vi "util_SwitchableDevice_cls_Turn On.vi"(0 "Interface_object in":refnum<class>, 5 "error in (no error)":errorcluster) -> (14 "Interface_object out":refnum<class>, 19 "error out":errorcluster)   [LabVIEW 2018, in "Lamp.lvclass"]
uses:
  Lamp.lvclass
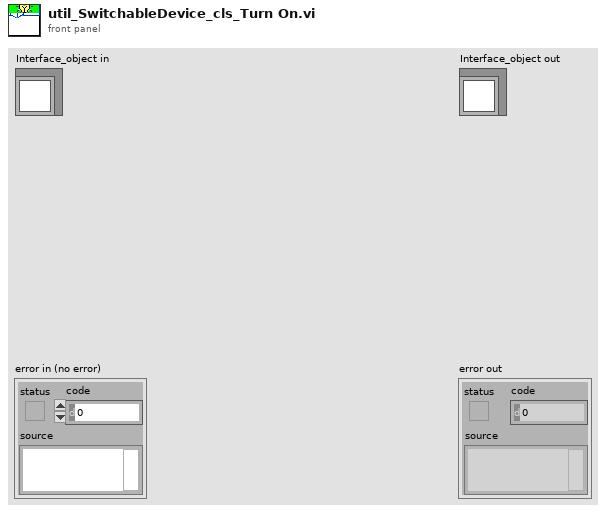
[diagram p1: front panel]
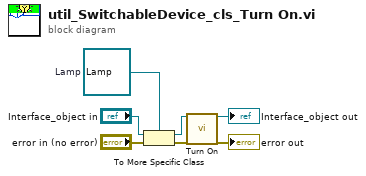
[diagram p0: block diagram]
diagram:
  w3 = refnum<class "Lamp.lvclass"> refnum  # Lamp
  n1 = To More Specific Class(target class=w3, reference="Interface_object in", error in="error in (no error)") -> (specific class reference=w1:refnum<class "Lamp.lvclass">, error out=w2:errorcluster)
  n2 = call-dynamic "Turn On.vi"("Interface_object in"=w1, "error in (no error)"=w2) -> ("Interface_object out"=→"Interface_object out":refnum<class "Lamp.lvclass">, "error out"=→"error out":errorcluster)  [unwired: 16 in]
